vi "工步列表.vi"(8 "Bool引用句柄":refnum<vi>, 9 "事件注册引用句柄 3":refnum<event-registration>, 10 "添加的数组 2":refnum<vi>[](array[refnum]), 11 "添加的数组":string[][][](array[string])) -> ()   [LabVIEW 2020]
uses:
  <vilib>/Utility/miscctls.llb/LVRectTypeDef.ctl
  Windows/System32/user32.dll
panel:
  in  "布尔 3":T1
  in  "布尔 2":T2
  in  "布尔":T3
  in  "树形控件":string(tree)
  # "工步数据"
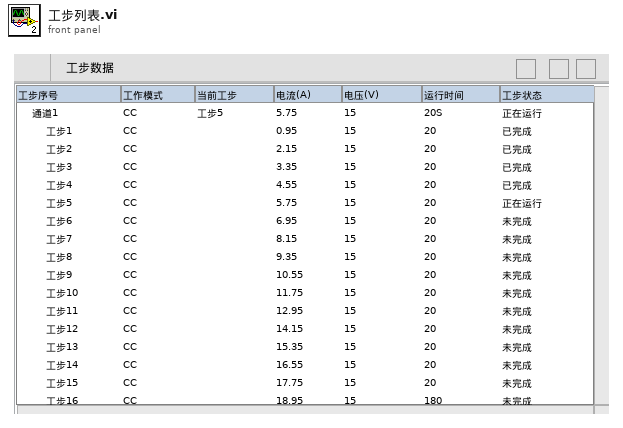
[diagram p1: front panel]
types:
  T1 = typedef "控件最小化.ctl" = bool
  T2 = typedef "控件最大化.ctl" = bool
  T3 = typedef "控件关闭.ctl" = bool
  T4 = typedef "LVRectTypeDef.ctl" = cluster{"Left":i16, "Top":i16, "Right":i16, "Bottom":i16}
  T5 = enum32{"Invalid", "Standard", "Closed", "Hidden", "Minimized", "Maximized"}
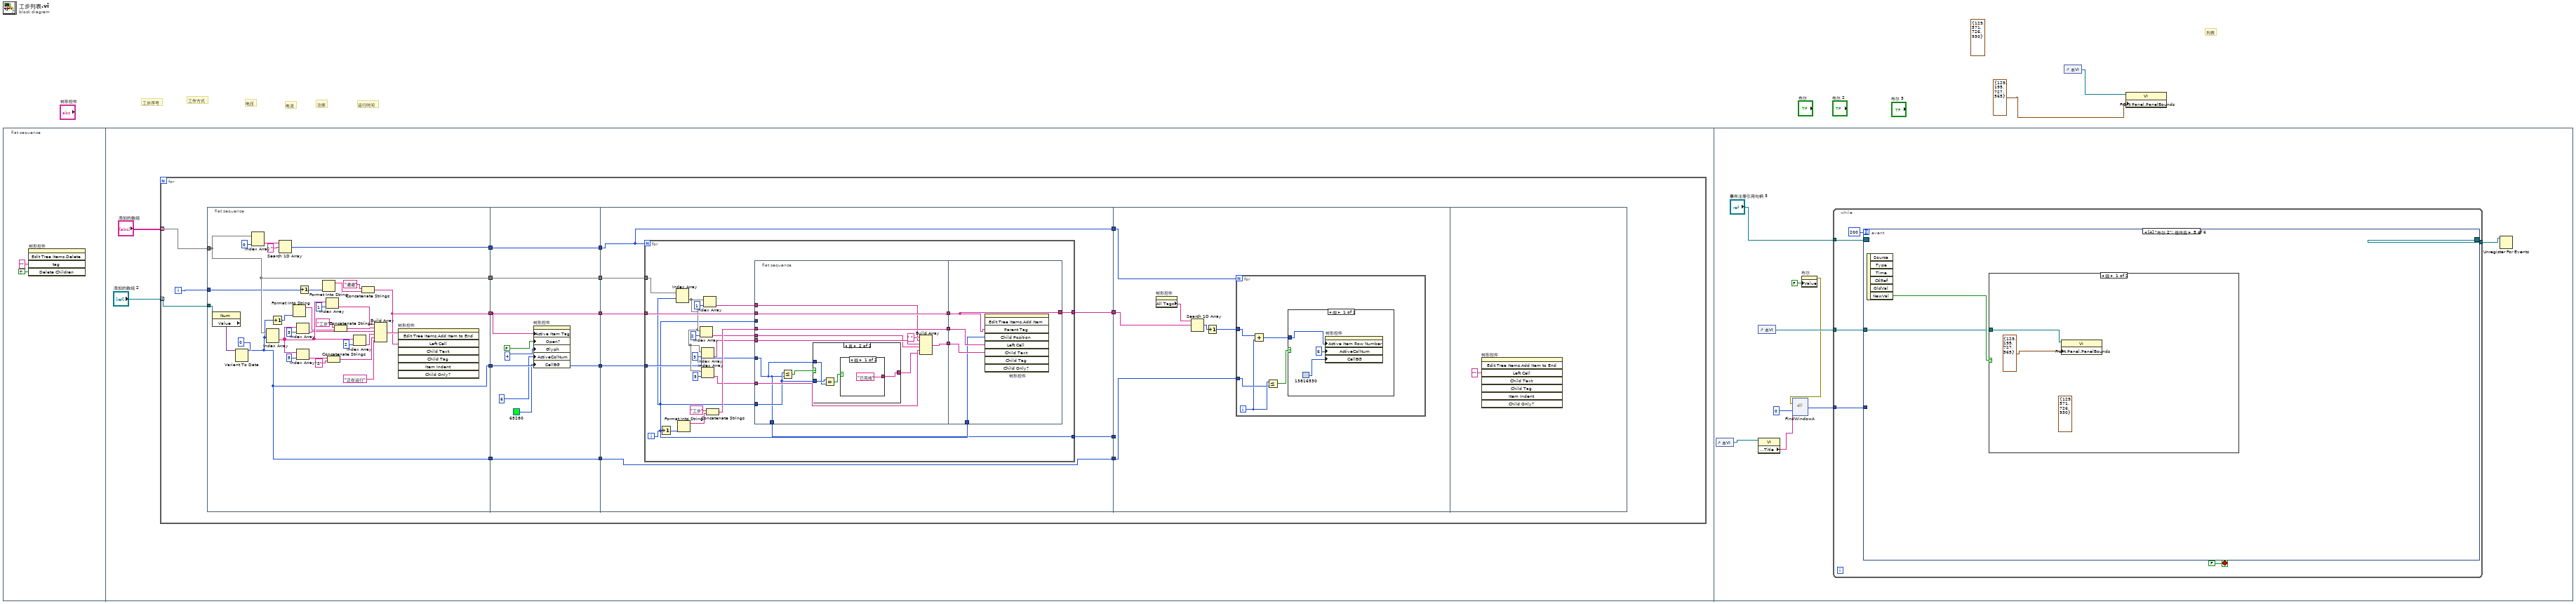
[diagram p0: block diagram]
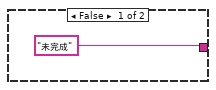
[diagram p2: hidden frame]
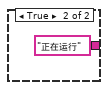
[diagram p3: hidden frame]
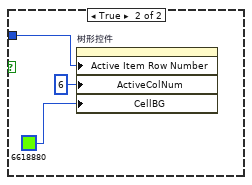
[diagram p4: hidden frame]
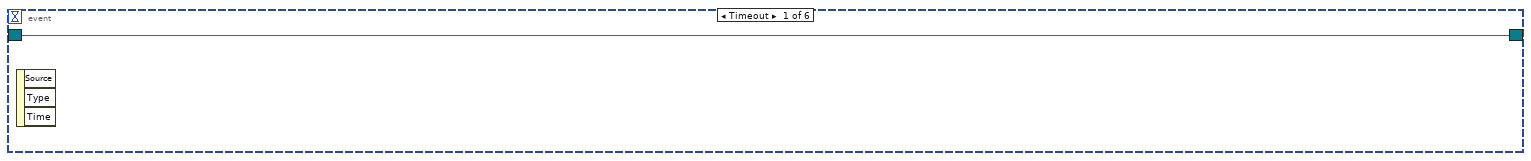
[diagram p5: hidden frame]
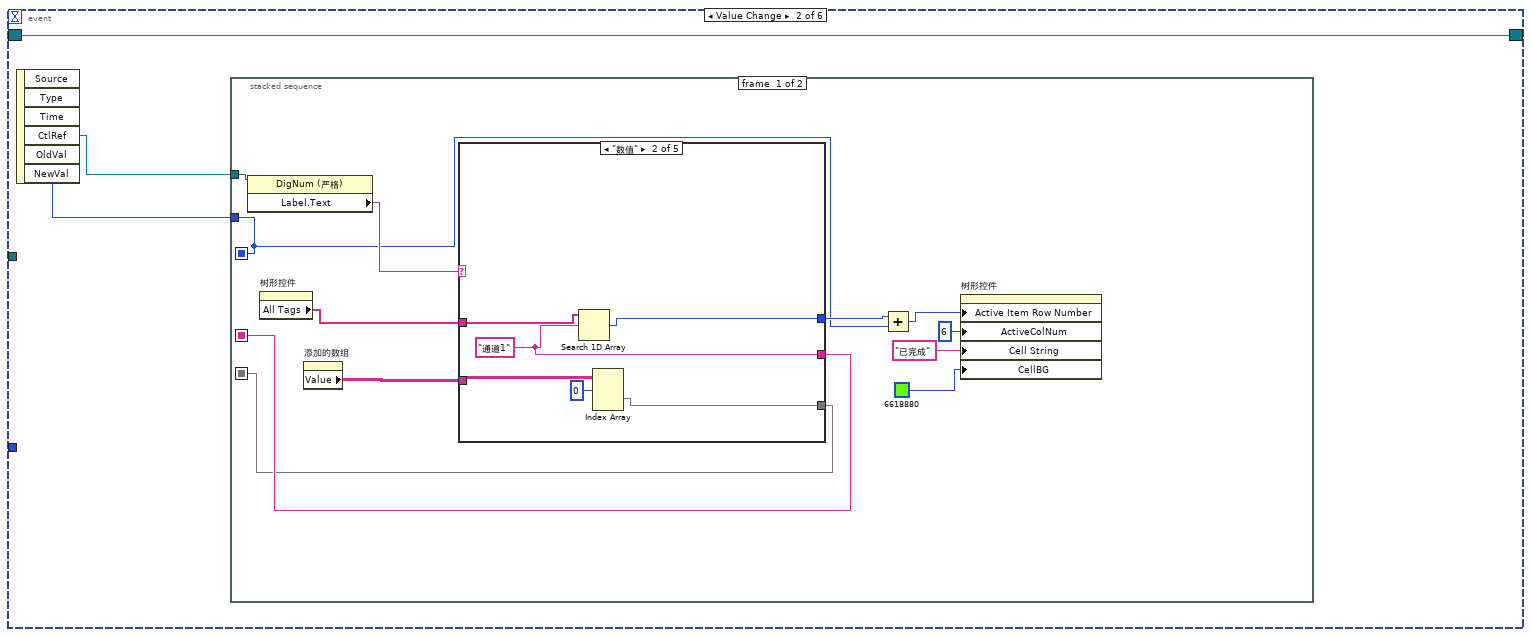
[diagram p6: hidden frame]
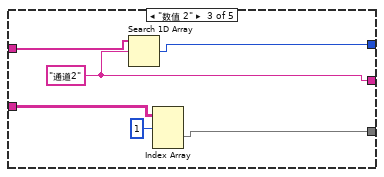
[diagram p8: hidden frame]
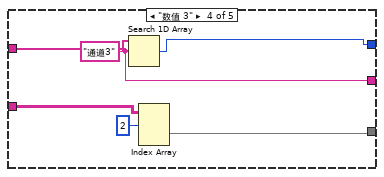
[diagram p9: hidden frame]
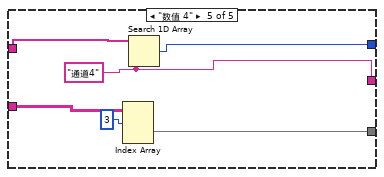
[diagram p10: hidden frame]
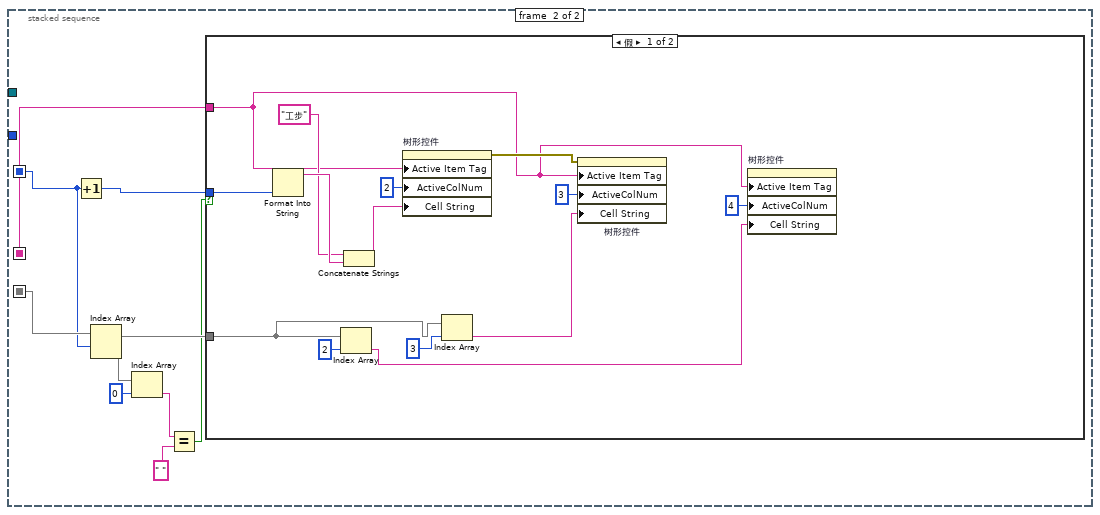
[diagram p11: hidden frame]
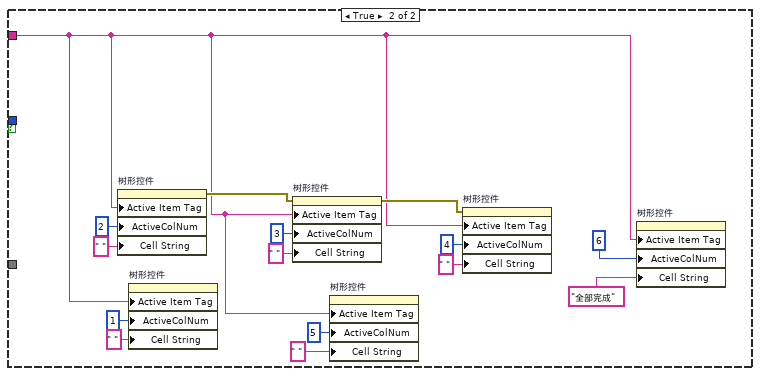
[diagram p12: hidden frame]
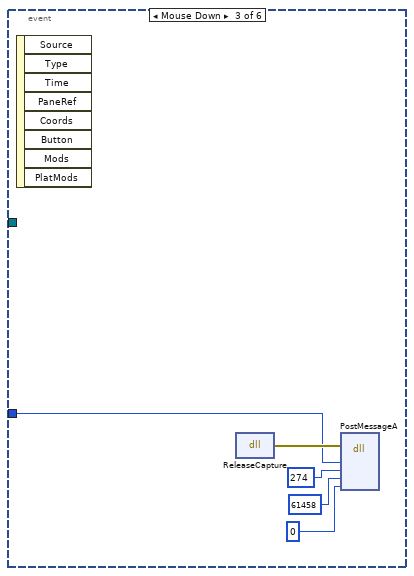
[diagram p13: hidden frame]
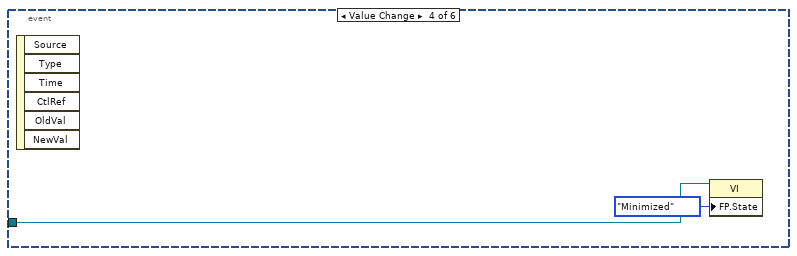
[diagram p14: hidden frame]
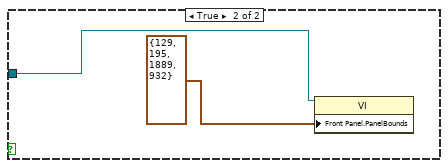
[diagram p15: hidden frame]
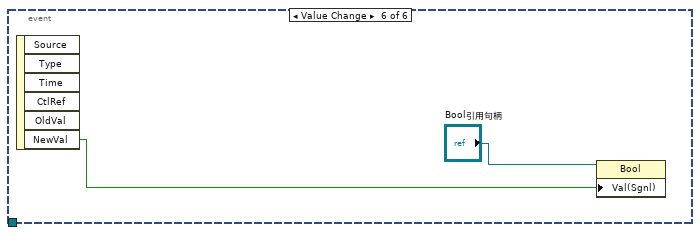
[diagram p16: hidden frame]
diagram:
  (unwired) T4 {"Left"=129, "Top"=571, "Right"=726, "Bottom"=930} ("前面板窗口:前面板边界")
  # "列表"
  # "运行时间"
  # "功率"
  # "电流"
  # "电压"
  # "工作方式"
  # "工步序号"
  n1 = flat-sequence {
    frame #0 {
      n2 = invoke on="树形控件" class="Tree (严格)" method="Edit Tree Items.Delete"("tag"="" ("标识符"), "Delete Children"=TRUE ("删除子项？")) -> ()  [unwired: 3 in, 5 out]
    }
    frame #1 {
      n3 = for {
        tunnel: "添加的数组" -> [w22] mode=indexing
        tunnel: "添加的数组 2" -> [w23] mode=indexing
        i -> [w7]
        n4 = flat-sequence {
          tunnel: w23 -> [w54]
          tunnel: w22 -> [w27]
          tunnel: [w28] -> w21
          tunnel: [w27] -> w19
          tunnel: [w26] -> w17
          tunnel: [w25] -> w15
          tunnel: [w25] -> w8
          tunnel: w7 -> [w24]
          tunnel: w21 -> [w63]
          tunnel: [w63] -> w20
          tunnel: w19 -> [w62]
          tunnel: [w62] -> w18
          tunnel: w17 -> [w60]
          tunnel: [w60] -> w16
          tunnel: w15 -> [w61]
          tunnel: [w61] -> w14
          tunnel: [w55] -> w9
          tunnel: w8 -> [w55]
          tunnel: w20 -> [w65]
          tunnel: w18 -> [w70]
          tunnel: w16 -> [w69]
          tunnel: w14 -> [w66]
          tunnel: [w68] -> w13
          tunnel: [w67] -> w12
          tunnel: [w65] -> w11
          tunnel: [w64] -> w10
          tunnel: w9 -> [w64]
          tunnel: w13 -> [_]
          tunnel: w12 -> [w120]
          tunnel: w11 -> [w117]
          tunnel: w10 -> [w116]
          frame #0 {
            n5 = property class="Num"(reference=w54) -> ("Value"=w48:variant)  [unwired: 1 in, 2 out]
            n6 = Variant To Data(type=0, Variant=w48) -> (data=w25:i32)  [unwired: 1 in, 1 out]
            n7 = Index Array(array=w27, index (col)=0 ("禁用的索引 (列)")) -> (element=w52:string[])  [unwired: 1 in]
            n8 = Index Array(array=w27, index (row)=w25) -> (element=w42:string[])  [unwired: 1 in]
            n9 = Increment(x=w25) -> (x+1=w29:i32)
            n10 = Search 1D Array(1D array=w52, element=" " ("元素")) -> (index of element=w28:i32)  [unwired: 1 in]
            n11 = Format Into String(w29) -> (resulting string=w39:string)  [unwired: 3 in, 1 out]
            n12 = Index Array(array=w42, index=3 ("索引")) -> (element=w37:string)
            n13 = Index Array(array=w42, index=5 ("索引")) -> (element=w33:string)
            n14 = Increment(x=w24) -> (x+1=w30:i32)
            n15 = Format Into String(w30) -> (resulting string=w49:string)  [unwired: 3 in, 1 out]
            n16 = Index Array(array=w42, index=1 ("索引")) -> (element=w41:string)
            n17 = Concatenate Strings(w33, "S" ("字符串")) -> (w31:string)
            n18 = Concatenate Strings("工步", w39) -> (w38:string)
            n19 = Index Array(array=w42, index=2 ("索引")) -> (element=w36:string)
            n20 = Concatenate Strings("通道", w49) -> (w26:string)
            n21 = Build Array(w41, w38, w37, w36, w31, "正在运行" ("元素")) -> (w34:string[])
            n22 = invoke on="树形控件" class="Tree (严格)" method="Edit Tree Items.Add Item to End"("Left Cell"=w26, "Child Text"=w34) -> ()  [unwired: 6 in, 8 out]
          }
          frame #1 {
            n23 = property on="树形控件" class="Tree (严格)"("Active Item Tag"=w60, "Open?"=FALSE ("活动项:打开？"), "Glyph"=4 ("活动项:符号索引"), "ActiveColNum"=6 ("活动单元格:活动列数"), "CellBG"=u32 65280) -> ()  [unwired: 2 in, 2 out]
          }
          frame #2 {
            n24 = for {
              N: w65 -> [_]
              tunnel: w70 -> [w91]
              tunnel: w69 -> [w90]
              tunnel: w66 -> [w81]
              tunnel: [w72] -> w68
              tunnel: [w71] -> w67
              i -> [w73]
              n25 = Increment(x=w73) -> (x+1=w92:i32)
              n26 = Index Array(array=w91, index (row)=w73) -> (element=w82:string[])  [unwired: 1 in]
              n27 = Format Into String(w92) -> (resulting string=w88:string)  [unwired: 3 in, 1 out]
              n28 = Index Array(array=w82, index=2 ("索引")) -> (element=w76:string)
              n29 = Index Array(array=w82, index=3 ("索引")) -> (element=w77:string)
              n30 = Index Array(array=w82, index=5 ("索引")) -> (element=w75:string)
              n31 = Index Array(array=w82, index=1 ("索引")) -> (element=w78:string)
              n32 = Concatenate Strings("工步" ("字符串"), w88) -> (w87:string)
              n33 = flat-sequence {
                tunnel: w90 -> [w102]
                tunnel: w73 -> [_]
                tunnel: w87 -> [w103]
                tunnel: w81 -> [w93]
                tunnel: w73 -> [w94]
                tunnel: [w103] -> w80
                tunnel: [w102] -> w79
                tunnel: w78 -> [w101]
                tunnel: w77 -> [w100]
                tunnel: w76 -> [w99]
                tunnel: w75 -> [w98]
                tunnel: [w96] -> w74
                tunnel: [w93] -> w72
                tunnel: w80 -> [w115]
                tunnel: w79 -> [w112]
                tunnel: w74 -> [w114]
                tunnel: w73 -> [w113]
                tunnel: [w112] -> w71
                frame #0 {
                  n34 = Less Or Equal?(x=w94, y=w93) -> (x <= y?=w104:bool)
                  n35 = case shown="真" w104 {
                    tunnel: ["未完成" w106] -> w97
                    tunnel: w94 -> [_ w109]
                    tunnel: w93 -> [_ w108]
                    frame False {
                    }
                    frame True {
                      n36 = Equal?(x=w109, y=w108) -> (x = y?=w107:bool)
                      n37 = case shown="假" w107 {
                        tunnel: ["已完成" "正在运行"] -> w106
                        frame False {
                        }
                        frame True {
                        }
                      }
                    }
                  }
                  n38 = Build Array(w101, " " ("元素"), w100, w99, w98, w97) -> (w96:string[])
                }
                frame #1 {
                  n39 = invoke on="树形控件" class="Tree (严格)" method="Edit Tree Items.Add Item"("Parent Tag"=w112, "Child Position"=w113, "Left Cell"=w115, "Child Text"=w114) -> ()  [unwired: 5 in, 9 out]
                }
              }
            }
          }
          frame #3 {
            n40 = property on="树形控件" class="Tree (严格)"() -> ("All Tags"=w121:string[])  [unwired: 2 in, 2 out]
            n41 = Search 1D Array(1D array=w121, element=w120) -> (index of element=w119:i32)  [unwired: 1 in]
            n42 = Increment(x=w119) -> (x+1=w118:i32)
            n43 = for {
              N: w117 -> [_]
              tunnel: w118 -> [w124]
              tunnel: w116 -> [w126]
              i -> [w123]
              n44 = Add(x=w124, y=w123) -> (x+y=w122:i32)
              n45 = Less Or Equal?(x=w123, y=w126) -> (x <= y?=w125:bool)
              n46 = case shown="假" w125 {
                tunnel: w122 -> [w127 w130]
                frame False {
                  n47 = property on="树形控件" class="Tree (严格)"("Active Item Row Number"=w127, "ActiveColNum"=6 ("活动单元格:活动列数"), "CellBG"=u32 13816530) -> ()  [unwired: 2 in, 2 out]
                }
                frame True {
                  n48 = property on="树形控件" class="Tree (严格)"("Active Item Row Number"=w130, "ActiveColNum"=6 ("活动单元格:活动列数"), "CellBG"=u32 6618880) -> ()  [unwired: 2 in, 2 out]
                }
              }
            }
          }
          frame #4 {
            n49 = invoke on="树形控件" class="Tree (严格)" method="Edit Tree Items.Add Item to End"("Left Cell"="" ("左单元格字符串")) -> ()  [unwired: 7 in, 8 out]
          }
        }
      }
    }
    frame #2 {
      n50 = control-ref of="本VI"() -> (w140:refnum<vi>)
      n51 = control-ref of="本VI"() -> (w137:refnum<vi>)
      n52 = property class="VI"(reference=w140) -> ("Front Panel.Title"=w141:string)  [unwired: 1 in, 2 out]
      n53 = property on="布尔" class="Bool (严格)"("Value"=T3 FALSE ("布尔")) -> (error out=w135:errorcluster)  [unwired: 2 in, 1 out]
      n54 = dll-call lib="/Windows/System32/user32.dll" fn="FindWindowA"(error in=w135, "lp"=u32 0, "name"=w141) -> ("返回类型"=w138:u32)  [unwired: 4 in, 2 out]
      n55 = while {
        tunnel: [w146] -> w142
        tunnel: w138 -> [w145]
        tunnel: w137 -> [w144]
        tunnel: "事件注册引用句柄 3" -> [w143]
        stop <- FALSE stop-if-true
        n56 = event shown="[4] \"布尔 2\": 值改变" {
          selector: w143 -> [w149 w152 _ _ _ _]
          dyn-events: [w149 w152 _ _ _ _] -> w146
          timeout: 200 -> [_ _ _ _ _ _]
          tunnel: w145 -> [_ _ w227 _ _ _]
          tunnel: w144 -> [_ _ _ w233 w234 _]
          event Timeout {
            n57 = event-data() -> ()  [unwired: 1 in, 3 out]
          }
          event Value Change {
            n58 = event-data() -> ("CtlRef"=w151:refnum<vi>, "NewVal"=w150:i32)  [unwired: 1 in, 4 out]
            n59 = stacked-sequence {
              seq-local: [w154 _] -> [_ w194]
              seq-local: [w158 _] -> [_ w195]
              seq-local: [w156 _] -> [_ w197]
              tunnel: w151 -> [w155 _]
              tunnel: w150 -> [w154 _]
              frame #0 {
                n60 = property class="DigNum (严格)"(reference=w155) -> ("Label.Text"=w164:string)  [unwired: 1 in, 2 out]
                n61 = property on="树形控件" class="Tree (严格)"() -> ("All Tags"=w163:string[])  [unwired: 2 in, 2 out]
                n62 = property on="添加的数组" class="Arr (严格)"() -> ("Value"=w157:string[][][])  [unwired: 2 in, 2 out]
                n63 = case shown="\"数值\"" w164 {
                  tunnel: w163 -> [_ w170 w176 w182 w188]
                  tunnel: [_ w169 w175 w181 w187] -> w162
                  tunnel: [_ w168 w174 w180 w186] -> w158
                  tunnel: w157 -> [_ w167 w173 w179 w185]
                  tunnel: [_ w165 w171 w177 w183] -> w156
                  frame "假", Default {
                  }
                  frame "数值" {
                    w168 = "通道1" ("元素")
                    n64 = Search 1D Array(1D array=w170, element=w168) -> (index of element=w169:i32)  [unwired: 1 in]
                    n65 = Index Array(array=w167, index (dim 0)=0 ("索引 (页)")) -> (element=w165:string[][])  [unwired: 2 in]
                  }
                  frame "数值 2" {
                    w174 = "通道2" ("元素")
                    n66 = Search 1D Array(1D array=w176, element=w174) -> (index of element=w175:i32)  [unwired: 1 in]
                    n67 = Index Array(array=w173, index (dim 0)=1 ("索引 (页)")) -> (element=w171:string[][])  [unwired: 2 in]
                  }
                  frame "数值 3" {
                    w180 = "通道3" ("元素")
                    n68 = Search 1D Array(1D array=w182, element=w180) -> (index of element=w181:i32)  [unwired: 1 in]
                    n69 = Index Array(array=w179, index (dim 0)=2 ("索引 (页)")) -> (element=w177:string[][])  [unwired: 2 in]
                  }
                  frame "数值 4" {
                    w186 = "通道4" ("元素")
                    n70 = Index Array(array=w185, index (dim 0)=3 ("索引 (页)")) -> (element=w183:string[][])  [unwired: 2 in]
                    n71 = Search 1D Array(1D array=w188, element=w186) -> (index of element=w187:i32)  [unwired: 1 in]
                  }
                }
                n72 = Add(x=w162, y=w154) -> (x+y=w161:i32)
                n73 = property on="树形控件" class="Tree (严格)"("Active Item Row Number"=w161, "ActiveColNum"=6 ("活动单元格:活动列数"), "Cell String"="已完成" ("活动单元格:字符串"), "CellBG"=u32 6618880) -> ()  [unwired: 2 in, 2 out]
              }
              frame #1 {
                n74 = Increment(x=w194) -> (x+1=w196:i32)
                n75 = Index Array(array=w197, index (row)=w194) -> (element=w193:string[])  [unwired: 1 in]
                n76 = Index Array(array=w193, index=0 ("索引")) -> (element=w191:string)
                n77 = Equal?(x=w191, y=" ") -> (x = y?=w189:bool)
                n78 = case shown="假" w189 {
                  tunnel: w196 -> [w207 _]
                  tunnel: w193 -> [w204 _]
                  tunnel: w195 -> [w200 w214]
                  frame False {
                    n79 = Format Into String(w207) -> (resulting string=w210:string)  [unwired: 3 in, 1 out]
                    n80 = Index Array(array=w204, index=2 ("索引")) -> (element=w198:string)
                    n81 = Concatenate Strings("工步" ("字符串"), w210) -> (w208:string)
                    n82 = property on="树形控件" class="Tree (严格)"("Active Item Tag"=w200, "ActiveColNum"=2 ("活动单元格:活动列数"), "Cell String"=w208) -> (error out=w203:errorcluster)  [unwired: 2 in, 1 out]
                    n83 = Index Array(array=w204, index=3 ("索引")) -> (element=w201:string)
                    n84 = property on="树形控件" class="Tree (严格)"(error in=w203, "Active Item Tag"=w200, "ActiveColNum"=3 ("活动单元格:活动列数"), "Cell String"=w201) -> ()  [unwired: 1 in, 2 out]
                    n85 = property on="树形控件" class="Tree (严格)"("Active Item Tag"=w200, "ActiveColNum"=4 ("活动单元格:活动列数"), "Cell String"=w198) -> ()  [unwired: 2 in, 2 out]
                  }
                  frame True {
                    n86 = property on="树形控件" class="Tree (严格)"("Active Item Tag"=w214, "ActiveColNum"=2 ("活动单元格:活动列数"), "Cell String"=" " ("活动单元格:字符串")) -> (error out=w223:errorcluster)  [unwired: 2 in, 1 out]
                    n87 = property on="树形控件" class="Tree (严格)"("Active Item Tag"=w214, "ActiveColNum"=1 ("活动单元格:活动列数"), "Cell String"=" " ("活动单元格:字符串")) -> ()  [unwired: 2 in, 2 out]
                    n88 = property on="树形控件" class="Tree (严格)"(error in=w223, "Active Item Tag"=w214, "ActiveColNum"=3 ("活动单元格:活动列数"), "Cell String"=" " ("活动单元格:字符串")) -> (error out=w224:errorcluster)  [unwired: 1 in, 1 out]
                    n89 = property on="树形控件" class="Tree (严格)"("Active Item Tag"=w214, "ActiveColNum"=5 ("活动单元格:活动列数"), "Cell String"=" " ("活动单元格:字符串")) -> ()  [unwired: 2 in, 2 out]
                    n90 = property on="树形控件" class="Tree (严格)"(error in=w224, "Active Item Tag"=w214, "ActiveColNum"=4 ("活动单元格:活动列数"), "Cell String"=" " ("活动单元格:字符串")) -> ()  [unwired: 1 in, 2 out]
                    n91 = property on="树形控件" class="Tree (严格)"("Active Item Tag"=w214, "ActiveColNum"=6 ("活动单元格:活动列数"), "Cell String"="全部完成" ("活动单元格:字符串")) -> ()  [unwired: 2 in, 2 out]
                  }
                }
              }
            }
          }
          event Mouse Down {
            n92 = event-data() -> ()  [unwired: 1 in, 8 out]
            n93 = dll-call lib="/Windows/System32/user32.dll" fn="ReleaseCapture"() -> (error out=w231:errorcluster)  [unwired: 4 in, 1 out]
            n94 = dll-call lib="/Windows/System32/user32.dll" fn="PostMessageA"(error in=w231, "lp"=w227, "name"=274, "vak"=61458, "val"=0) -> ()  [unwired: 7 in, 2 out]
          }
          event Value Change {
            n95 = event-data() -> ()  [unwired: 1 in, 6 out]
            n96 = property class="VI"(reference=w233, "FP.State"=T5."Minimized" ("前面板窗口:状态")) -> ()  [unwired: 1 in, 2 out]
          }
          event Value Change {
            n97 = event-data() -> ("NewVal"=w235:T2)  [unwired: 1 in, 5 out]
            n98 = case shown="假" w235 {
              tunnel: w234 -> [w237 w238]
              frame False {
                (unwired) T4 {"Left"=129, "Top"=571, "Right"=726, "Bottom"=930} ("前面板窗口:前面板边界")
                n99 = property class="VI"(reference=w237, "Front Panel.PanelBounds"=T4 {"Left"=129, "Top"=195, "Right"=727, "Bottom"=565} ("前面板窗口:前面板边界")) -> ()  [unwired: 1 in, 2 out]
              }
              frame True {
                n100 = property class="VI"(reference=w238, "Front Panel.PanelBounds"=T4 {"Left"=129, "Top"=195, "Right"=1889, "Bottom"=932} ("前面板窗口:前面板边界")) -> ()  [unwired: 1 in, 2 out]
              }
            }
          }
          event Value Change {
            n101 = event-data() -> ("NewVal"=w240:T3)  [unwired: 1 in, 5 out]
            n102 = property class="Bool"(reference="Bool引用句柄", "Val(Sgnl)"=w240) -> ()  [unwired: 1 in, 2 out]
          }
        }
      }
      n103 = Unregister For Events(event registration refnum=w142) -> ()  [unwired: 1 in, 1 out]
    }
  }
  n104 = control-ref of="本VI"() -> (w2:refnum<vi>)
  n105 = property class="VI"(reference=w2, "Front Panel.PanelBounds"=T4 {"Left"=129, "Top"=195, "Right"=727, "Bottom"=565} ("前面板窗口:前面板边界")) -> ()  [unwired: 1 in, 2 out]
